vi "Begin routeguide_RouteGuide_ListFeatures.vi"(8 "error in":errorcluster, 10 "Request Data":T1, 11 "gRPC ID":T3) -> (0 "error out":errorcluster, 2 "Call Id Out":T3, 3 "gRPC ID out":T3)   [LabVIEW 2019, in "route_guide_client.lvlib"]
uses:
  route_guide_client.lvlib
  <vilib>/gRPC/LabVIEW gRPC Library/Shared/grpcId.ctl
  RPC Messages/routeguide_Rectangle.ctl
  RPC Messages/routeguide_Point.ctl
  59bd46bd-855a-43b3-a0b3-6a244c6a481b.vi
  <vilib>/gRPC/LabVIEW gRPC Library/Server API/Server/Get Server DLL Path.vi
  <vilib>/gRPC/LabVIEW gRPC Library/Shared/TranslateGrpcError.vi
  <vilib>/gRPC/LabVIEW gRPC Library/gprc-lvsupport-release.lvlib
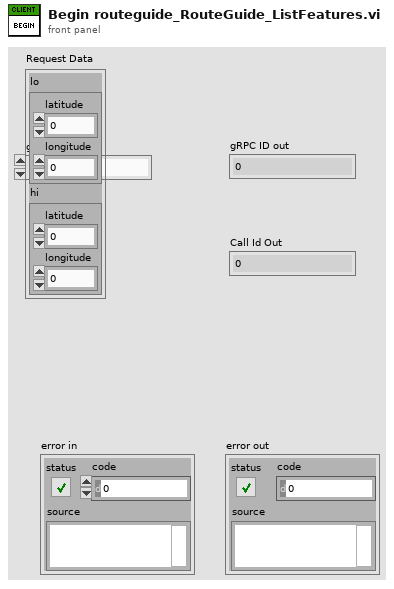
[diagram p1: front panel]
types:
  T1 = typedef "route_guide_client.lvlib/routeguide_Rectangle.ctl" = cluster{"lo":T2, "hi":T2}
  T2 = typedef "route_guide_client.lvlib/routeguide_Point.ctl" = cluster{"latitude":i32, "longitude":i32}
  T3 = typedef "gprc-lvsupport-release.lvlib/grpcId.ctl" = u64
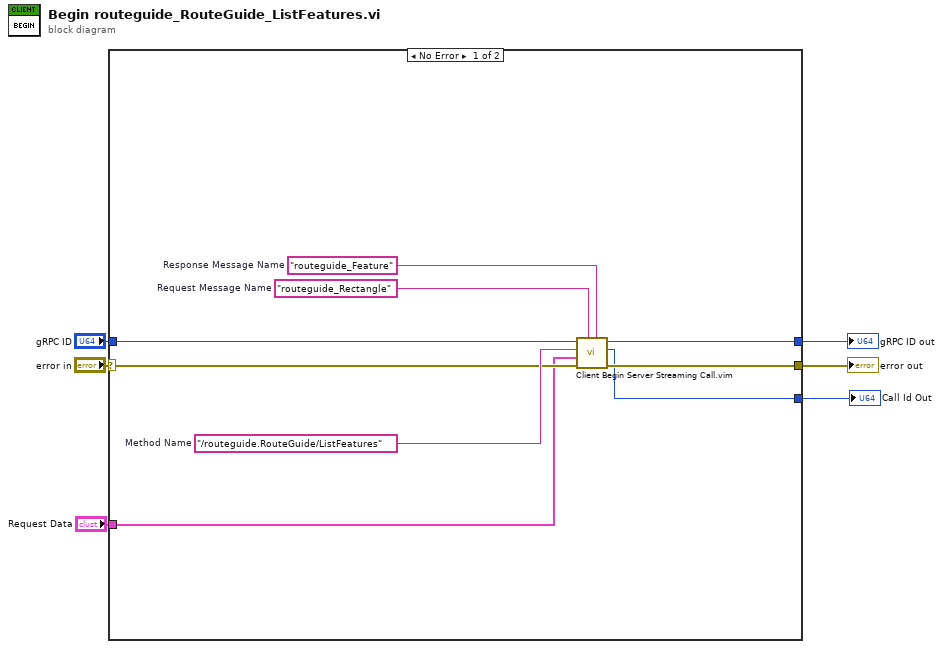
[diagram p0: block diagram]
diagram:
  n1 = case shown="No Error" "error in" {
    selector: "error in" -> [w12 w16]
    tunnel: [w11 w16] -> w5
    tunnel: "gRPC ID" -> [w10 w17]
    tunnel: [w9 w17] -> w3
    tunnel: [w8 _] -> w2
    tunnel: "Request Data" -> [w7 _]
    frame No Error {
      w13 = "routeguide_Feature"  # Response Message Name
      w14 = "routeguide_Rectangle"  # Request Message Name
      w15 = "/routeguide.RouteGuide/ListFeatures"  # Method Name
      n2 = call "Client Begin Server Streaming Call.vim"("Response Message Name"=w13, "Request Message Name"=w14, "error in"=w12, "Request Data"=w7, "Method Name"=w15, "ClientID in"=w10) -> ("error out"=w11:errorcluster, "Call ID out"=w8:u64, "ClientID out"=w9:u64)  [unwired: 3 in]
    }
    frame Error {
    }
  }
  "error out" <- w5
  "gRPC ID out" <- w3
  "Call Id Out" <- w2
